vi "FileStream Flush.vi"(8 "error in (no error)":errorcluster, 11 "reference":refnum<k24>) -> (0 "error out":errorcluster, 3 "reference out":refnum<k24>)   [LabVIEW 2017, in "File Stream.lvlib"]
doc: "Clears buffers for this stream and causes any buffered data to be written to the file, and also clears all intermediate file buffers."
uses:
  File Stream.lvlib
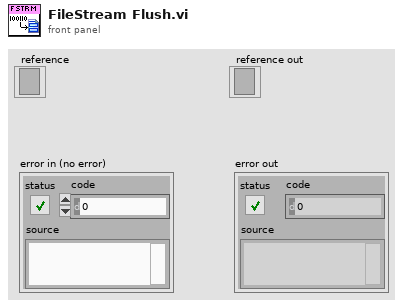
[diagram p1: front panel]
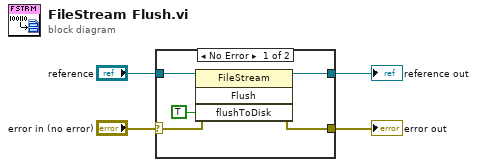
[diagram p0: block diagram]
diagram:
  n1 = case shown="No Error" "error in (no error)" {
    selector: "error in (no error)" -> [w8 w10]
    tunnel: "reference" -> [w9 w11]
    tunnel: [w7 w11] -> w2
    tunnel: [w6 w10] -> w1
    frame No Error {
      n2 = invoke class="FileStream" method="Flush"(reference=w9, error in=w8, "flushToDisk"=TRUE) -> (reference out=w7:refnum<k24>, error out=w6:errorcluster)  [unwired: 1 in, 2 out]
    }
    frame Error {
    }
  }
  "reference out" <- w2
  "error out" <- w1
